vi "WPI_UtilitiesGetTreeIOName.vi"(10 "NewVal":string, 11 "TreeControl in":refnum<vi>) -> (3 "I/O Name":string)   [LabVIEW 2017]
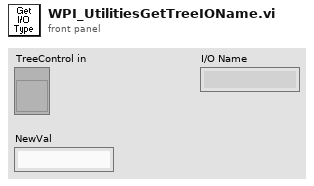
[diagram p1: front panel]
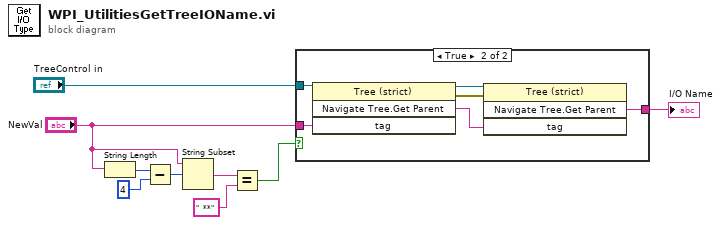
[diagram p0: block diagram]
diagram:
  n1 = String Length(string="NewVal") -> (length=w7:i32)
  n2 = Subtract(x=w7, y=4) -> (x-y=w8:i32)
  n3 = String Subset(string="NewVal", offset (0)=w8) -> (substring=w4:string)  [unwired: 1 in]
  n4 = Equal?(x=w4, y="  **") -> (x = y?=w2:bool)
  n5 = case shown="True" w2 {
    tunnel: "TreeControl in" -> [_ w15]
    tunnel: "NewVal" -> [_ w11]
    tunnel: [_ w10] -> w1
    frame False {
    }
    frame True {
      n6 = invoke class="Tree (strict)" method="Navigate Tree.Get Parent"(reference=w15, "tag"=w11) -> (reference out=w14:refnum<vi>, error out=w12:errorcluster, "Navigate Tree:Get Parent"=w13:string)  [unwired: 2 in, 1 out]
      n7 = invoke class="Tree (strict)" method="Navigate Tree.Get Parent"(reference=w14, error in=w12, "tag"=w13) -> ("Navigate Tree:Get Parent"=w10:string)  [unwired: 1 in, 3 out]
    }
  }
  "I/O Name" <- w1
